vi "IsPointIntoBounds.vi"(8 "error in (no error)":errorcluster, 10 "Point":dbl[](array[numeric]), 11 "object in":refnum<class "Zone.lvclass">) -> (0 "error out":errorcluster, 2 "IntoBounds":bool, 3 "object out":refnum<class "Zone.lvclass">)   [LabVIEW 2023, in "Zone.lvclass"]
uses:
  Zone.lvclass
  Game_class/Game.lvclass
  Zone.lvclass/Zone.ctl
  Utilities_class/Utilities.lvclass
panel:
  in  "Game":refnum<class "Game.lvclass">
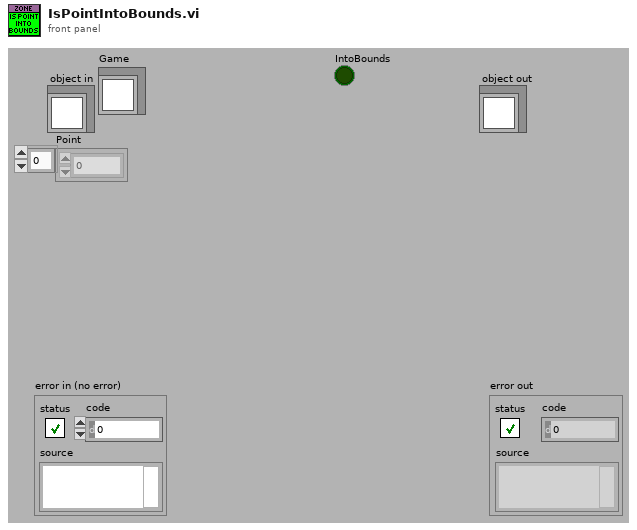
[diagram p1: front panel]
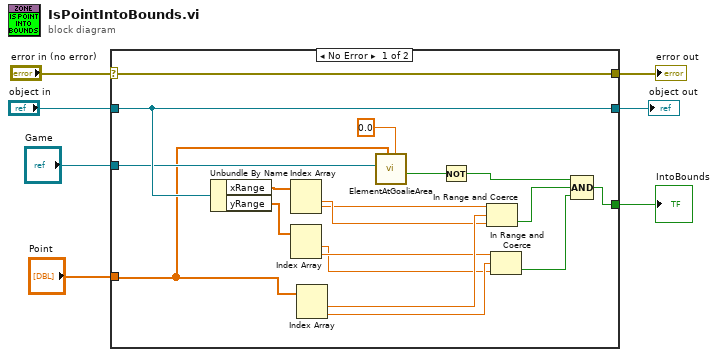
[diagram p0: block diagram]
diagram:
  n1 = case shown="No Error" "error in (no error)" {
    selector: "error in (no error)" -> [w25 w27]
    tunnel: [w25 w27] -> w6
    tunnel: [w24 w26] -> w4
    tunnel: "object in" -> [w24 w26]
    tunnel: "Point" -> [w9 _]
    tunnel: [w12 _] -> w2
    tunnel: "Game" -> [w11 _]
    frame No Error {
      n2 = Unbundle By Name(w24) -> ("xRange"=w21:dbl[], "yRange"=w20:dbl[])
      n3 = Index Array(array=w21) -> (element #1=w19:dbl, element #2=w18:dbl)  [unwired: 2 in]
      n4 = Index Array(array=w20) -> (element #1=w16:dbl, element #2=w17:dbl)  [unwired: 2 in]
      n5 = Index Array(array=w9) -> (element #1=w23:dbl, element #2=w22:dbl)  [unwired: 2 in]
      n6 = call "ElementAtGoalieArea.vi"("ElementRadius"=0.0, "Elemento pos."=w9, "Game"=w11) -> ("Element at our goalkeeper area ?"=w10:bool)  [unwired: 4 in, 4 out]
      n7 = Not(x=w10) -> (.not. x?=w13:bool)
      n8 = In Range and Coerce(upper limit=w18, x=w23, lower limit=w19) -> (In Range?=w15:bool)  [unwired: 1 out]
      n9 = In Range and Coerce(upper limit=w17, x=w22, lower limit=w16) -> (In Range?=w14:bool)  [unwired: 1 out]
      n10 = Compound Arithmetic op=AND(w13, w15, w14) -> (w12:bool)
    }
    frame Error {
    }
  }
  "error out" <- w6
  "object out" <- w4
  "IntoBounds" <- w2
